vi "Create.vi"(4 "Node":string, 6 "System":string, 8 "error in (no error)":errorcluster, 10 "Unconfigured":bool) -> (0 "error out":errorcluster, 3 "HomeHTTPController out":refnum<class "HomeHTTPController.lvclass">)   [LabVIEW 2020, in "Volatus.lvlib" / "HomeHTTPController.lvclass"]
uses:
  HomeHTTPController.lvclass
  HomeHTTPController.lvclass/HomeHTTPController.ctl
  HTTP Nav.ctl
  Volatus.lvlib
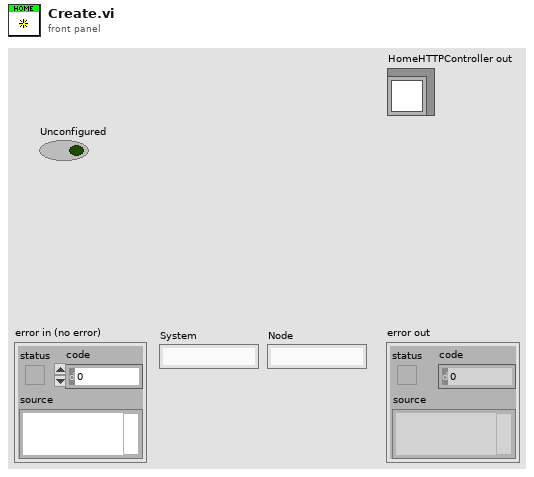
[diagram p1: front panel]
types:
  T1 = typedef "Volatus.lvlib/HTTP Nav.ctl" = cluster{"Name":string, "Path":string}
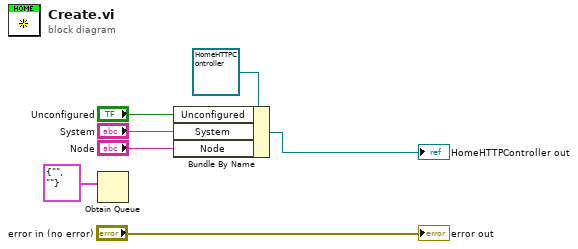
[diagram p0: block diagram]
diagram:
  n1 = Obtain Queue(element data type=T1 {"Name"="", "Path"=""} ("HTTP Nav")) -> ()  [unwired: 4 in, 3 out]
  n2 = Bundle By Name(cluster=refnum<class "HomeHTTPController.lvclass"> refnum ("HomeHTTPController in"), "Unconfigured"="Unconfigured", "System"="System", "Node"="Node") -> (→"HomeHTTPController out":refnum<class "HomeHTTPController.lvclass">)
  "error out" <- "error in (no error)"
